vi "CheckForFileFolders.vi"(0 "Main Path":path, 5 "Sub Path":string[](array[string]), 11 "Error in (no error)":errorcluster, 13 "Operation":enum16{"Create Files", "Create Folders"}(ring)=enum."Create Folders") -> (4 "Array":path[](array[path]), 15 "Error out":errorcluster)   [LabVIEW 2017]
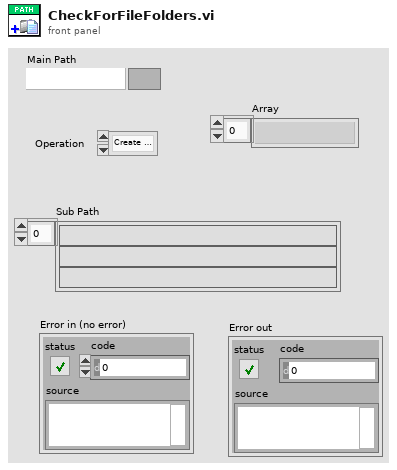
[diagram p1: front panel]
types:
  T1 = enum16{"open", "replace", "create", "open or create", "replace or create", "replace or create with confirmation"}
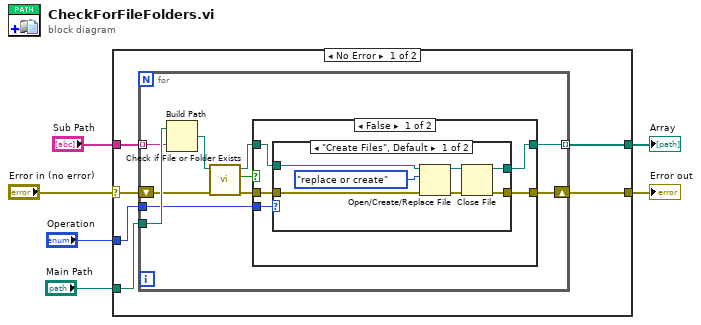
[diagram p0: block diagram]
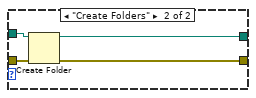
[diagram p2: hidden frame]
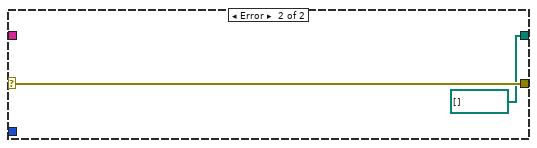
[diagram p4: hidden frame]
diagram:
  n1 = case shown="No Error" "Error in (no error)" {
    selector: "Error in (no error)" -> [w7 w42]
    tunnel: "Sub Path" -> [w12 _]
    tunnel: "Main Path" -> [w11 _]
    tunnel: "Operation" -> [w10 _]
    tunnel: [w9 path[] []] -> w3
    tunnel: [w8 w42] -> w2
    frame No Error {
      n2 = for {
        tunnel: w11 -> [w22]
        tunnel: w12 -> [w21] mode=indexing
        tunnel: [w15] -> w9 mode=indexing
        tunnel: w10 -> [w13]
        shift-right: [w14] -> w8
        shift-left: w7 -> [w17]
        n3 = Build Path(base path=w22, name or relative path=w21) -> (appended path=w20:path)
        n4 = call <vilib>:"Check if File or Folder Exists.vi"("error in (no error)"=w17, "path"=w20) -> ("error out"=w18:errorcluster, "file or folder exists?"=w19:bool, "dup path"=w16:path)  [unwired: 7 in]
        n5 = case shown="False" w19 {
          tunnel: w18 -> [w27 w39]
          tunnel: [w26 w39] -> w14
          tunnel: w16 -> [w25 w40]
          tunnel: [w24 w40] -> w15
          tunnel: w13 -> [w23 _]
          frame False {
            n6 = case shown="\"Create Files\", Default" w23 {
              tunnel: w27 -> [w34 w38]
              tunnel: [w30 w37] -> w26
              tunnel: w25 -> [w32 w36]
              tunnel: [w28 w35] -> w24
              frame "Create Files", Default {
                n7 = Open/Create/Replace File(file path (use dialog)=w32, error in=w34, operation (0:open)=T1."replace or create") -> (refnum out=w29:refnum<file>, error out=w31:errorcluster)  [unwired: 3 in, 1 out]
                n8 = Close File(refnum=w29, error in=w31) -> (path=w28:path, error out=w30:errorcluster)
              }
              frame "Create Folders" {
                n9 = Create Folder(path (use dialog)=w36, error in=w38) -> (created path=w35:path, error out=w37:errorcluster)  [unwired: 1 in, 1 out]
              }
            }
          }
          frame True {
          }
        }
      }
    }
    frame Error {
    }
  }
  "Array" <- w3
  "Error out" <- w2
